vi "RS232c.vi"() -> ()   [LabVIEW 2015]
uses:
  <vilib>/Instr/_visa.llb/VISA Configure Serial Port (Instr).vi
  <instrlib>/Agilent 532XX Series/Public/Data/Low Level/Fetch Measurement (Single).vi
  <instrlib>/Agilent 532XX Series/Agilent 532XX Series.lvlib
panel:
  out "Ph = ADAM-4017, CH3 [ V ]:":string
  out "Ph = ADAM-4017, CH4 [ V ]:":string
  out "Pl = ADAM-4017, CH2 [ V ]:":string
  out "Ph = ADAM-4017, CH1 [ V ]:":string
  out "Read Buffer 1 ADAM-4017: 5":dbl
  out "Read Buffer 1 ADAM-4017: 4":dbl
  out "Write Buffer 1 ADAM-4017: 5":dbl
  out "Write Buffer 1 ADAM-4017: 4":dbl
  out "Read Buffer 1 ADAM-4017: 3":dbl
  out "Write Buffer 1 ADAM-4017: 3":dbl
  out "Read Buffer 1 ADAM-4017: 2":dbl
  out "Write Buffer 1 ADAM-4017: 2":dbl
  out "Tiempo 2":dbl
  in  "stop 2":bool
  in  "Tab Control":enum32{"CONFIGURATION", "ERROR"}(tab)
  out "?":dbl
  out "Humidity[ppm]":dbl
  out "Substance 1[ppm]":dbl
  out "Substance 2[ppm]":dbl
  in  "ENABLE CONFIGURATION":bool
  in  "baud rate (9600)":u32=115200
  in  "data bits (8)":u16=8 min=5 max=8 step=1
  in  "parity (0:none)":u16(ring) items=["None", "Odd", "Even", "Mark", "Space"]
  in  "flow control":u16(ring) items=["None"=0, "XON/XOFF"=1, "RTS/CTS"=2, "DTR/DSR"=4]
  in  "VISA resource name (write)":refnum<visa-resource-name>="COM1"
  in  "stop bits":u16(ring)=10 items=["1.0"=10, "1.5"=15, "2.0"=20]
  in  "Voltios":dbl
  out "output string":string
  out "output string 3":string
  in  "Voltios 2":dbl
  out "output string 4":string
  in  "Voltios 3":dbl
  out "output string 5":string
  in  "Voltios 4":dbl
  in  "VISA resource name":refnum<visa-resource-name>
  in  "Timeout (10000 ms)":u32=10000
  out "Measurement":dbl format="%#_12g"
  out "Canal 4":cluster{dbl[], dbl[]}(graph) caption="Temperatura SAW"
  out "Ph = ADAM-4017, CH1 [ V ]:":string
  out "Ph = ADAM-4017, CH2 [ V ]:":string
  out "Ph = ADAM-4017, CH4 [ V ]:":string
  out "Ph = ADAM-4017, CH5 [ V ]:":string
  out "Write Buffer 1 ADAM-4017:":dbl
  out "Read Buffer 1 ADAM-4017:":dbl
  out "Write Buffer 2 ADAM-4017:":dbl
  out "Read Buffer 2 ADAM-4017:":dbl
  out "Write Buffer 3 ADAM-4017:":dbl
  out "Read Buffer 3 ADAM-4017:":dbl
  out "Read Buffer 4 ADAM-4017:":dbl
  out "Write Buffer 4 ADAM-4017:":dbl
  in  "error in (no error)":errorcluster
  out "error out":errorcluster
  out "VISA resource name out":refnum<visa-resource-name>
  out "Time:":string="00:00:00"
  out "Date:":string="01-01-2010"
  out "bytes written 5":u32=1
  out "bytes written 4":u32=1
  out "bytes written 3":u32=1
  out "bytes written 2":u32=1
  out "output string 2":string
  out "return count":u32
  out "Serial Settings:Number of Bytes at Serial Port":u32
  out "unsigned byte array 2":u8[](array[numeric])
  out "read buffer":string
  out "bytes written":u32=1
  # "WRITE"
  # "Air [ppm]"
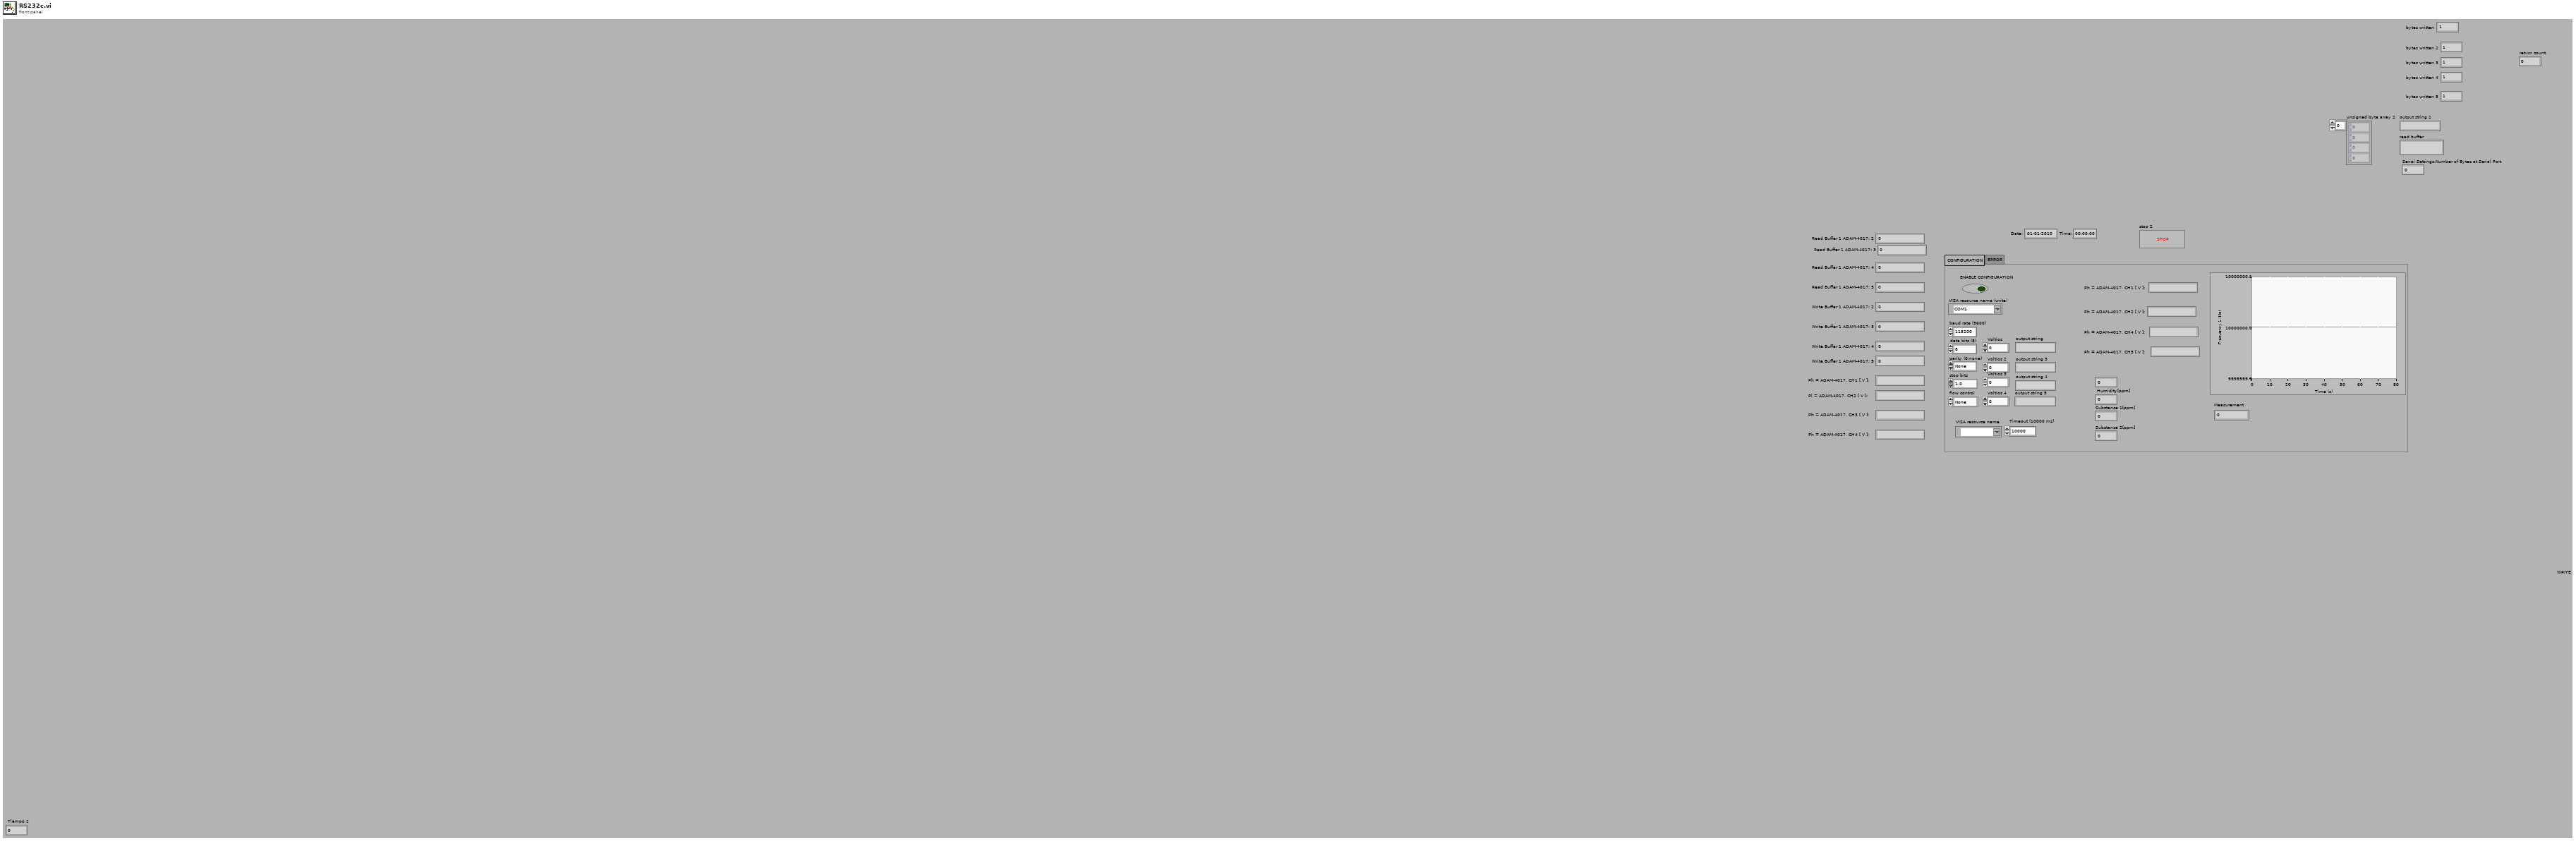
[diagram p1: front panel]
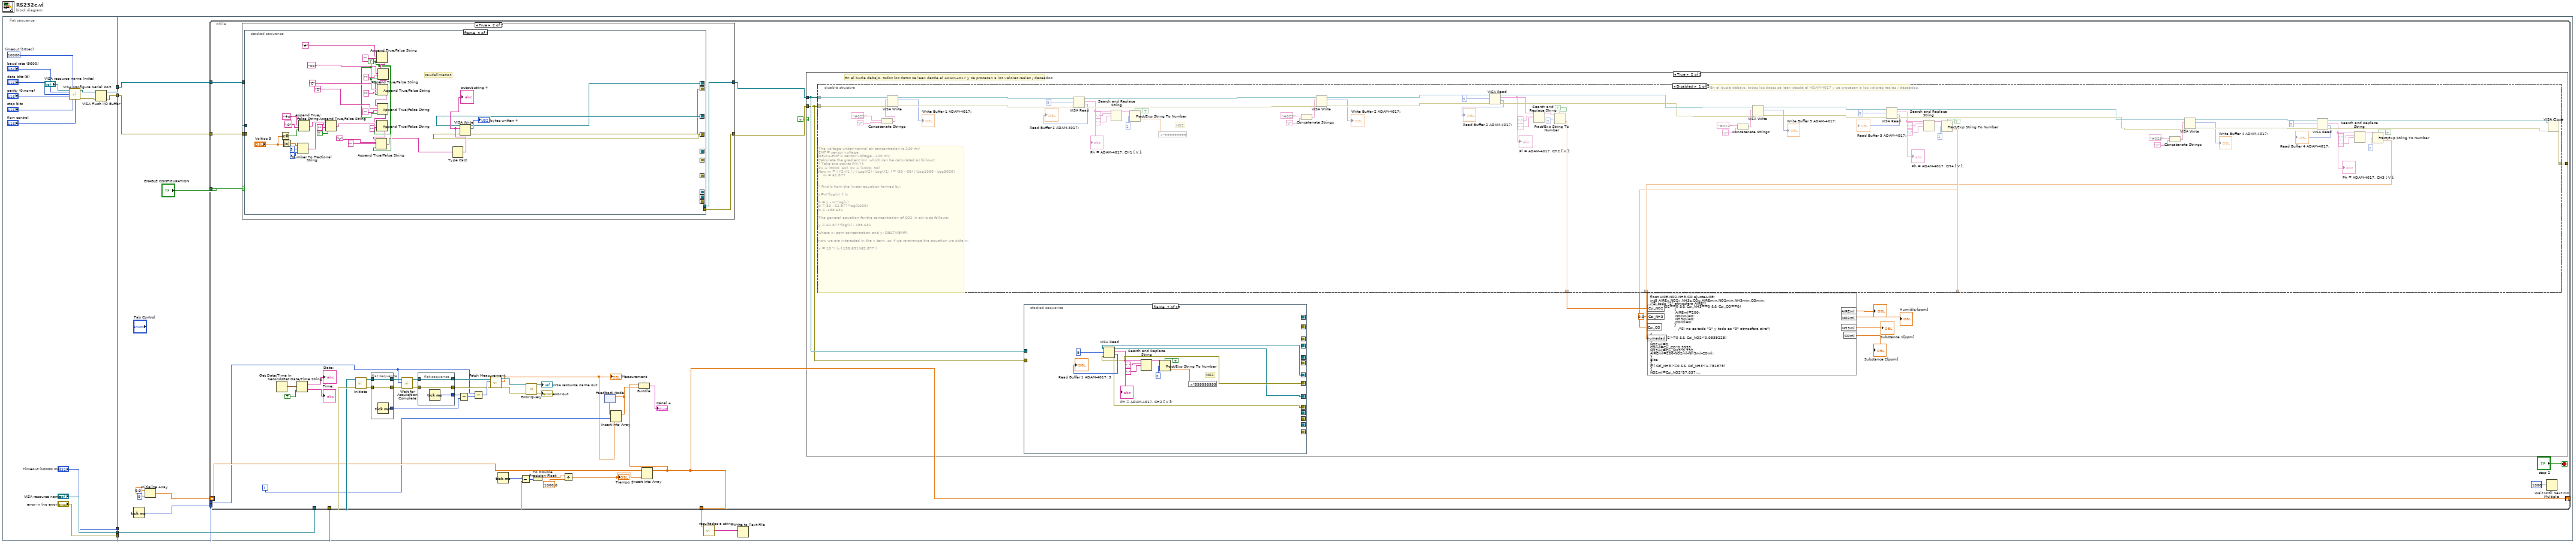
[diagram p0: block diagram]
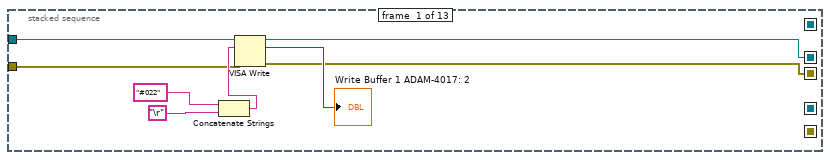
[diagram p4: hidden frame]
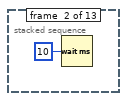
[diagram p5: hidden frame]
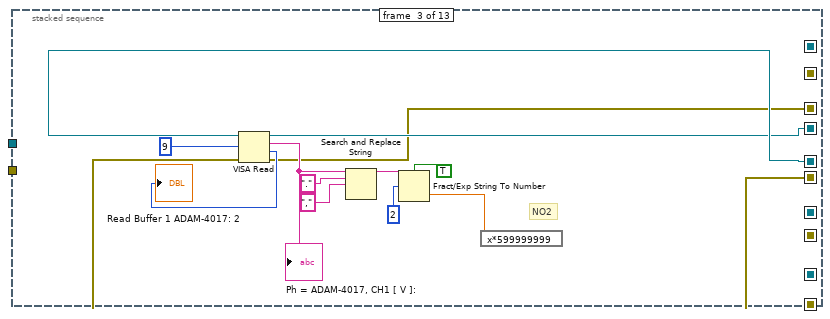
[diagram p6: hidden frame]
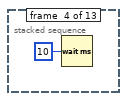
[diagram p7: hidden frame]
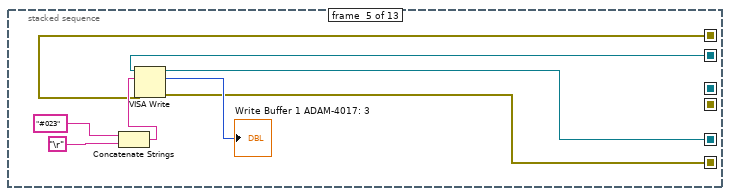
[diagram p8: hidden frame]
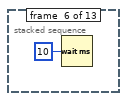
[diagram p9: hidden frame]
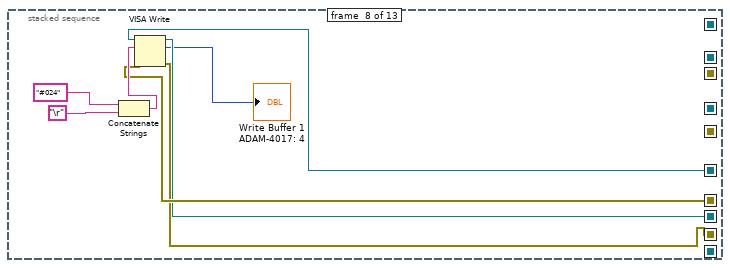
[diagram p10: hidden frame]
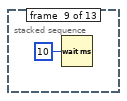
[diagram p11: hidden frame]
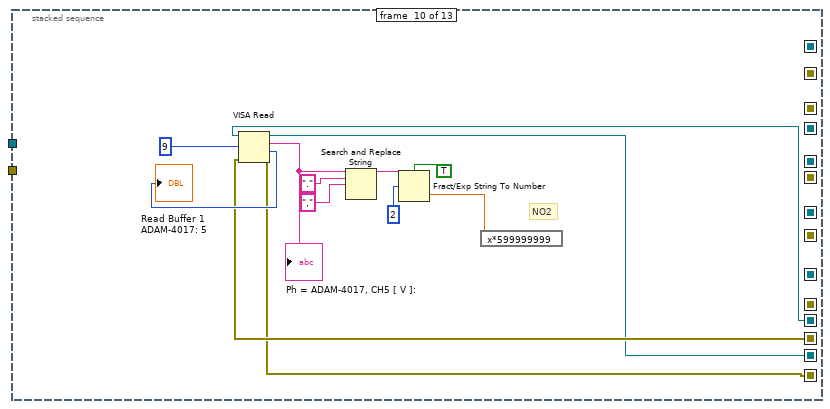
[diagram p12: hidden frame]
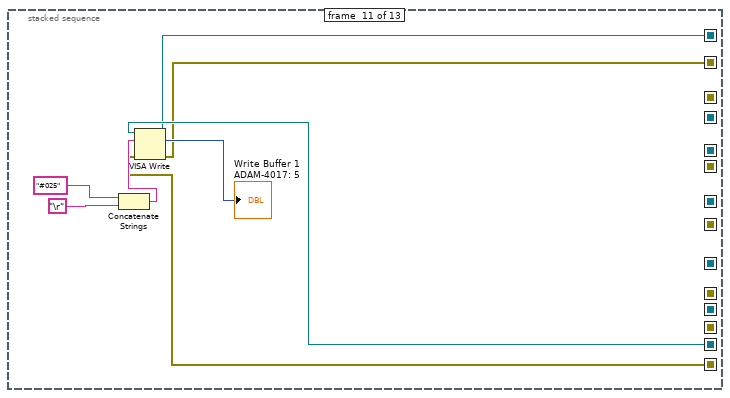
[diagram p13: hidden frame]
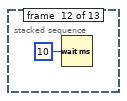
[diagram p14: hidden frame]
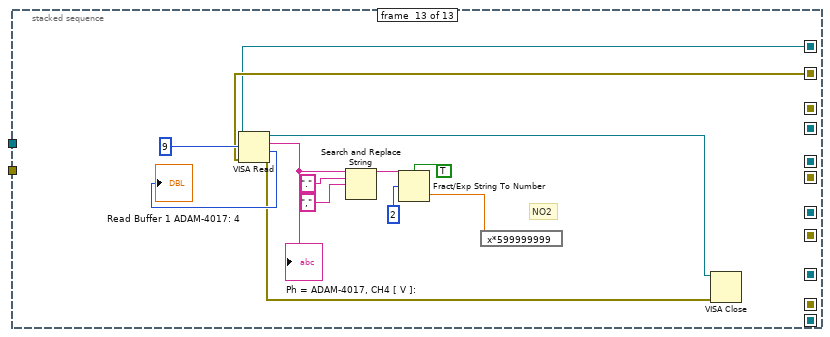
[diagram p15: hidden frame]
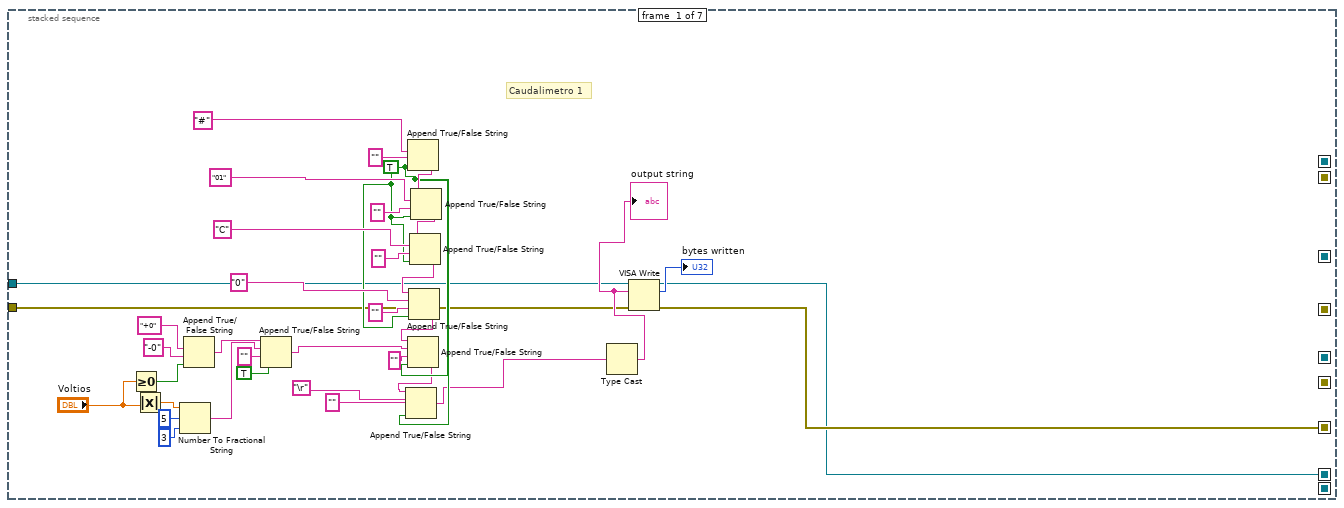
[diagram p17: hidden frame]
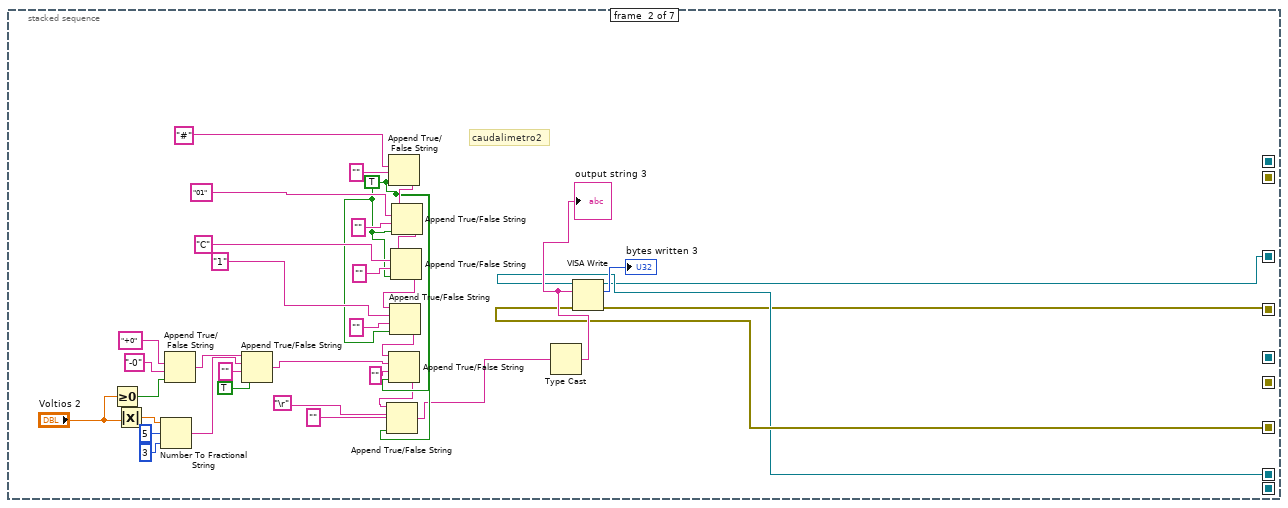
[diagram p18: hidden frame]
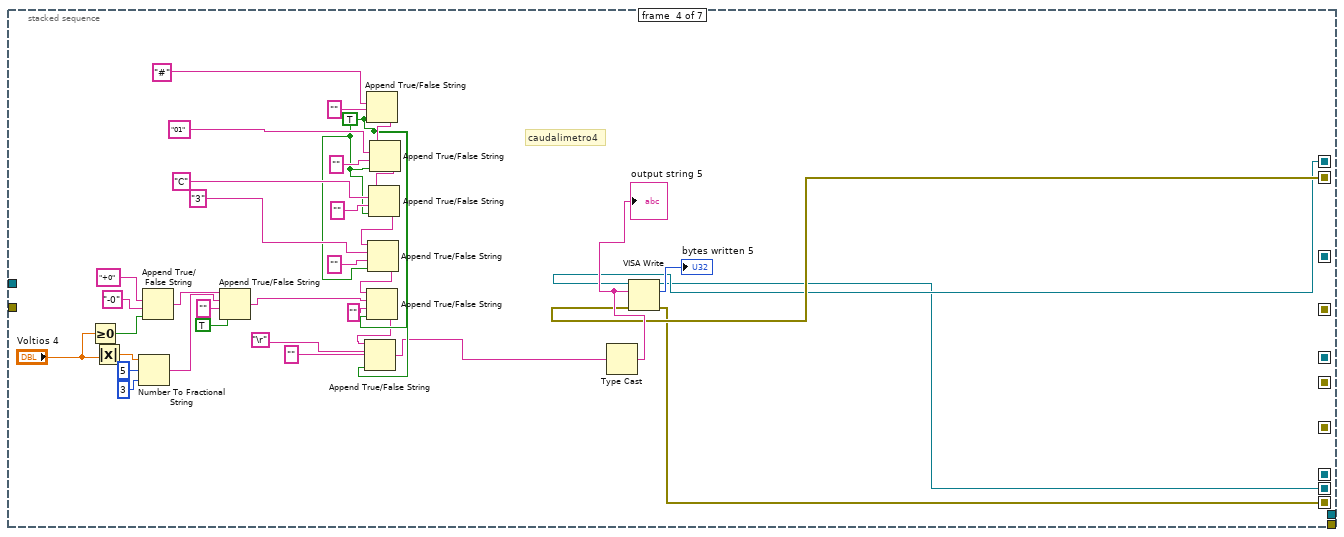
[diagram p19: hidden frame]
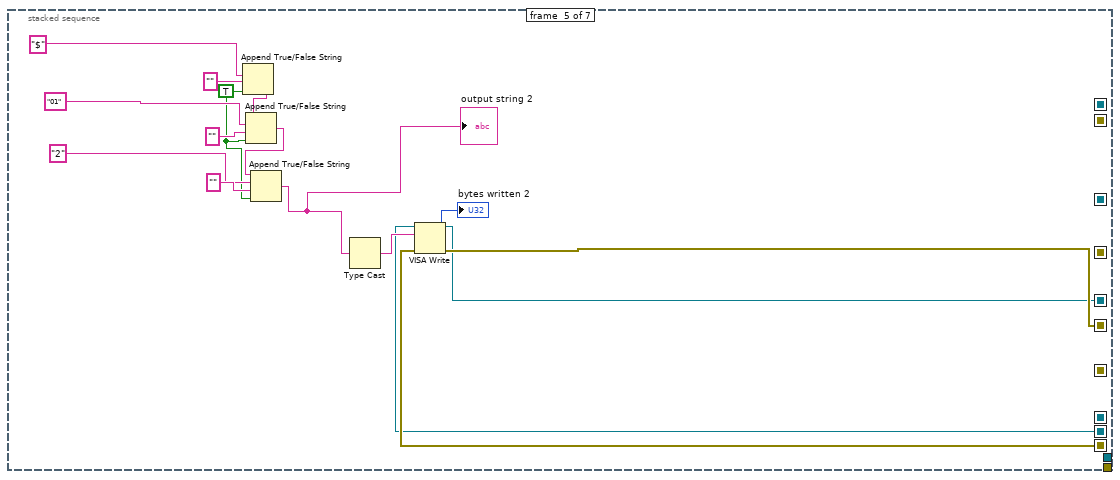
[diagram p20: hidden frame]
diagram:
  n1 = flat-sequence {
    tunnel: [w10] -> w5
    tunnel: [w9] -> w4
    tunnel: ["error in (no error)"] -> w3
    tunnel: ["VISA resource name"] -> w2
    tunnel: ["Timeout (10000 ms)"] -> w1
    tunnel: w5 -> [w31]
    tunnel: w4 -> [w30]
    tunnel: w3 -> [w28]
    tunnel: w2 -> [w27]
    tunnel: w1 -> [w26]
    frame #0 {
      w12 = u32 10000  # timeout (10sec)
      n2 = call-poly "VISA Configure Serial Port"("VISA resource name"="VISA resource name (write)", "timeout (10sec)"=w12, "baud rate (9600)"="baud rate (9600)", "data bits (8)"="data bits (8)", "parity (0:none)"="parity (0:none)", "stop bits (10: 1 bit)"="stop bits", "flow control (0:none)"="flow control") -> ("VISA resource name out"=w18:refnum<visa-resource-name>, "error out"=w19:errorcluster)  [unwired: 7 in]
      n3 = VISA Flush I/O Buffer(VISA resource name=w18, error in (no error)=w19) -> (VISA resource name out=w9:refnum<visa-resource-name>, error out=w10:errorcluster)  [unwired: 1 in]
    }
    frame #1 {
      n4 = Tick Count (ms)() -> (millisecond timer value=w25:u32)
      n5 = Initialize Array(0.0 ("element"), 0 ("dimension size")) -> (w22:dbl[])
      n6 = while {
        tunnel: w31 -> [w75]
        tunnel: w30 -> [w74]
        tunnel: "ENABLE CONFIGURATION" -> [w73]
        tunnel: w28 -> [w47]
        tunnel: w27 -> [w46]
        tunnel: w26 -> [w32]
        shift-right: [w33] -> _
        shift-left: w22 -> [w40]
        tunnel: w25 -> [w39]
        tunnel: [w33] -> w20
        i -> [w37]
        stop <- "stop 2" stop-if-true
        n7 = case shown="True" w73 {
          tunnel: w75 -> [w255 w259]
          tunnel: w74 -> [w254 w258]
          tunnel: [w255 w257] -> w72
          tunnel: [w254 w256] -> w71
          frame False {
          }
          frame True {
            n8 = stacked-sequence {
              seq-local: [w294 _ _ _ _ _ _] -> [_ w299 _ _ _ _ _]
              seq-local: [w293 _ _ _ _ _ _] -> [_ w298 _ _ _ _ _]
              seq-local: [_ _ _ _ w410 _ _] -> [_ _ _ _ _ _ w426]
              seq-local: [_ _ _ _ w409 _ _] -> [_ _ _ _ _ _ w425]
              seq-local: [_ w297 _ _ _ _ _] -> [_ _ w334 _ _ _ _]
              seq-local: [_ w296 _ _ _ _ _] -> [_ _ w335 _ _ _ _]
              seq-local: [_ _ w333 _ _ _ _] -> [_ _ _ w371 _ _ _]
              seq-local: [_ _ w332 _ _ _ _] -> [_ _ _ w370 _ _ _]
              seq-local: [_ _ _ w368 _ _ _] -> [_ _ _ _ w405 _ _]
              seq-local: [_ _ _ w369 _ _ _] -> [_ _ _ _ w406 _ _]
              tunnel: w259 -> [w261 _ _ _ _ _ _]
              tunnel: w258 -> [w260 _ _ _ _ _ _]
              tunnel: [_ _ _ _ _ _ w422] -> w257
              tunnel: [_ _ _ _ _ _ w421] -> w256
              frame #0 {
                w279 = TRUE ("selector")
                # "Caudalimetro 1"
                n9 = Greater Or Equal To 0?(x="Voltios") -> (x >= 0?=w267:bool)
                n10 = Absolute Value(x="Voltios") -> (abs(x)=w265:dbl)
                n11 = Number To Fractional String(number=w265, width (-)=i16 5, precision (6)=i16 3) -> (F-format string=w271:string)  [unwired: 1 in]
                n12 = Append True/False String(1:w267, 2:"-0" ("false string"), 3:"+0") -> (0:w272:string)  [unwired: 1 in]
                n13 = Append True/False String(1:TRUE ("selector"), 2:"" ("false string"), 3:w271, 4:w272) -> (0:w266:string)
                n14 = Append True/False String(1:w279, 2:"" ("false string"), 3:"#") -> (0:w287:string)  [unwired: 1 in]
                n15 = Append True/False String(1:w279, 2:"" ("false string"), 3:"01" ("INI"), 4:w287) -> (0:w286:string)
                n16 = Append True/False String(1:w279, 2:"" ("false string"), 3:"C" ("MASK"), 4:w286) -> (0:w292:string)
                n17 = Append True/False String(1:w279, 2:"" ("false string"), 3:"0" ("Canal"), 4:w292) -> (0:w280:string)
                n18 = Append True/False String(1:w279, 2:"", 3:w266, 4:w280) -> (0:w277:string)
                n19 = Append True/False String(1:w279, 2:"" ("false string"), 3:"\r", 4:w277) -> (0:w263:string)
                n20 = Type Cast(x=w263) -> (*(type *) &x=w262:string)  [unwired: 1 in]
                "output string" <- w262
                n21 = VISA Write(VISA resource name=w260, write buffer=w262, error in (no error)=w261) -> (VISA resource name out=w293:refnum<visa-resource-name>, return count=→"bytes written":u32, error out=w294:errorcluster)
              }
              frame #1 {
                w317 = TRUE ("selector")
                # "caudalimetro2"
                n22 = Greater Or Equal To 0?(x="Voltios 2") -> (x >= 0?=w305:bool)
                n23 = Absolute Value(x="Voltios 2") -> (abs(x)=w303:dbl)
                n24 = Number To Fractional String(number=w303, width (-)=i16 5, precision (6)=i16 3) -> (F-format string=w309:string)  [unwired: 1 in]
                n25 = Append True/False String(1:w305, 2:"-0" ("false string"), 3:"+0") -> (0:w310:string)  [unwired: 1 in]
                n26 = Append True/False String(1:TRUE ("selector"), 2:"" ("false string"), 3:w309, 4:w310) -> (0:w304:string)
                n27 = Append True/False String(1:w317, 2:"" ("false string"), 3:"#") -> (0:w325:string)  [unwired: 1 in]
                n28 = Append True/False String(1:w317, 2:"" ("false string"), 3:"01" ("INI"), 4:w325) -> (0:w324:string)
                n29 = Append True/False String(1:w317, 2:"" ("false string"), 3:"C" ("MASK"), 4:w324) -> (0:w330:string)
                n30 = Append True/False String(1:w317, 2:"" ("false string"), 3:"1" ("Canal 2"), 4:w330) -> (0:w318:string)
                n31 = Append True/False String(1:w317, 2:"", 3:w304, 4:w318) -> (0:w315:string)
                n32 = Append True/False String(1:w317, 2:"" ("false string"), 3:"\r", 4:w315) -> (0:w301:string)
                n33 = Type Cast(x=w301) -> (*(type *) &x=w300:string)  [unwired: 1 in]
                "output string 3" <- w300
                n34 = VISA Write(VISA resource name=w298, write buffer=w300, error in (no error)=w299) -> (VISA resource name out=w296:refnum<visa-resource-name>, return count=→"bytes written 3":u32, error out=w297:errorcluster)
              }
              frame #2 {
                w353 = TRUE ("selector")
                # "caudalimetro3"
                n35 = Greater Or Equal To 0?(x="Voltios 3") -> (x >= 0?=w341:bool)
                n36 = Absolute Value(x="Voltios 3") -> (abs(x)=w339:dbl)
                n37 = Number To Fractional String(number=w339, width (-)=i16 5, precision (6)=i16 3) -> (F-format string=w345:string)  [unwired: 1 in]
                n38 = Append True/False String(1:w341, 2:"-0" ("false string"), 3:"+0") -> (0:w346:string)  [unwired: 1 in]
                n39 = Append True/False String(1:TRUE ("selector"), 2:"" ("false string"), 3:w345, 4:w346) -> (0:w340:string)
                n40 = Append True/False String(1:w353, 2:"" ("false string"), 3:"#") -> (0:w361:string)  [unwired: 1 in]
                n41 = Append True/False String(1:w353, 2:"" ("false string"), 3:"01" ("INI"), 4:w361) -> (0:w360:string)
                n42 = Append True/False String(1:w353, 2:"" ("false string"), 3:"C" ("MASK"), 4:w360) -> (0:w366:string)
                n43 = Append True/False String(1:w353, 2:"" ("false string"), 3:"2" ("Canal 3"), 4:w366) -> (0:w354:string)
                n44 = Append True/False String(1:w353, 2:"", 3:w340, 4:w354) -> (0:w351:string)
                n45 = Append True/False String(1:w353, 2:"" ("false string"), 3:"\r", 4:w351) -> (0:w337:string)
                n46 = Type Cast(x=w337) -> (*(type *) &x=w336:string)  [unwired: 1 in]
                "output string 4" <- w336
                n47 = VISA Write(VISA resource name=w335, write buffer=w336, error in (no error)=w334) -> (VISA resource name out=w332:refnum<visa-resource-name>, return count=→"bytes written 4":u32, error out=w333:errorcluster)
              }
              frame #3 {
                w389 = TRUE ("selector")
                # "caudalimetro4"
                n48 = Greater Or Equal To 0?(x="Voltios 4") -> (x >= 0?=w377:bool)
                n49 = Absolute Value(x="Voltios 4") -> (abs(x)=w375:dbl)
                n50 = Number To Fractional String(number=w375, width (-)=i16 5, precision (6)=i16 3) -> (F-format string=w381:string)  [unwired: 1 in]
                n51 = Append True/False String(1:w377, 2:"-0" ("false string"), 3:"+0") -> (0:w382:string)  [unwired: 1 in]
                n52 = Append True/False String(1:TRUE ("selector"), 2:"" ("false string"), 3:w381, 4:w382) -> (0:w376:string)
                n53 = Append True/False String(1:w389, 2:"" ("false string"), 3:"#") -> (0:w397:string)  [unwired: 1 in]
                n54 = Append True/False String(1:w389, 2:"" ("false string"), 3:"01" ("INI"), 4:w397) -> (0:w396:string)
                n55 = Append True/False String(1:w389, 2:"" ("false string"), 3:"C" ("MASK"), 4:w396) -> (0:w402:string)
                n56 = Append True/False String(1:w389, 2:"" ("false string"), 3:"3" ("Canal 4"), 4:w402) -> (0:w390:string)
                n57 = Append True/False String(1:w389, 2:"", 3:w376, 4:w390) -> (0:w387:string)
                n58 = Append True/False String(1:w389, 2:"" ("false string"), 3:"\r", 4:w387) -> (0:w373:string)
                n59 = Type Cast(x=w373) -> (*(type *) &x=w372:string)  [unwired: 1 in]
                "output string 5" <- w372
                n60 = VISA Write(VISA resource name=w370, write buffer=w372, error in (no error)=w371) -> (VISA resource name out=w368:refnum<visa-resource-name>, return count=→"bytes written 5":u32, error out=w369:errorcluster)
              }
              frame #4 {
                w408 = TRUE ("selector")
                n61 = Append True/False String(1:w408, 2:"" ("false string"), 3:"$") -> (0:w415:string)  [unwired: 1 in]
                n62 = Append True/False String(1:w408, 2:"" ("false string"), 3:"01" ("INI"), 4:w415) -> (0:w414:string)
                n63 = Append True/False String(1:w408, 2:"" ("false string"), 3:"2" ("MASK"), 4:w414) -> (0:w404:string)
                "output string 2" <- w404
                n64 = Type Cast(x=w404) -> (*(type *) &x=w407:string)  [unwired: 1 in]
                n65 = VISA Write(VISA resource name=w405, write buffer=w407, error in (no error)=w406) -> (VISA resource name out=w409:refnum<visa-resource-name>, return count=→"bytes written 2":u32, error out=w410:errorcluster)
              }
              frame #5 {
                n66 = Wait (ms)(milliseconds to wait=u32 1000) -> ()  [unwired: 1 out]
              }
              frame #6 {
                n67 = property class="Instr"(reference=w425, error in=w426) -> (reference out=w431:refnum<visa-resource-name>, error out=w430:errorcluster, "Bytes at Port"=w429:u32)
                "Serial Settings:Number of Bytes at Serial Port" <- w429
                n68 = VISA Read(VISA resource name=w431, byte count=w429, error in (no error)=w430) -> (VISA resource name out=w421:refnum<visa-resource-name>, read buffer=w424:string, return count=→"return count":u32, error out=w422:errorcluster)
                n69 = String To Byte Array(string=w424) -> (unsigned byte array=→"unsigned byte array 2":u8[])
                n70 = Type Cast(x=w424) -> (*(type *) &x=→"read buffer":string)  [unwired: 1 in]
              }
            }
          }
        }
        n71 = Get Date/Time In Seconds() -> (seconds since 1Jan1904=w67:timestamp)
        n72 = Get Date/Time String(seconds (now)=w67, want seconds? (F)=TRUE) -> (date string=→"Date:":string, time string=→"Time:":string)  [unwired: 1 in]
        n73 = call <instrlib>:"Initiate.vi"("error in (no error)"=w47, "VISA resource name"=w46) -> ("error out"=w59:errorcluster, "VISA resource name out"=w60:refnum<visa-resource-name>)  [unwired: 8 out]
        n74 = flat-sequence {
          tunnel: [w81] -> w56
          tunnel: w60 -> [w81]
          tunnel: [w80] -> w57
          tunnel: w59 -> [w80]
          tunnel: [w79] -> w58
          frame #0 {
            n75 = Tick Count (ms)() -> (millisecond timer value=w79:u32)
          }
        }
        n76 = call <instrlib>:"Wait for Acquisition Complete.vi"("error in (no error)"=w57, "Maximum Time (10000 ms)"=w32, "VISA resource name"=w56) -> ("error out"=w54:errorcluster, "VISA resource name out"=w55:refnum<visa-resource-name>)  [unwired: 1 in, 6 out]
        n77 = flat-sequence {
          tunnel: [w78] -> w50
          tunnel: w55 -> [w78]
          tunnel: [w77] -> w51
          tunnel: w54 -> [w77]
          tunnel: [w76] -> w53
          frame #0 {
            n78 = Tick Count (ms)() -> (millisecond timer value=w76:u32)
          }
        }
        n79 = Subtract(x=w53, y=w58) -> (x-y=w61:u32)
        n80 = Subtract(x=w32, y=w61) -> (x-y=w52:u32)
        n81 = call-poly <instrlib>:"Fetch Measurement.vi"("error in (no error)"=w51, "Timeout (10000 ms)"=w52, "VISA resource name"=w50) -> ("error out"=w48:errorcluster, "Measurement"=w35:dbl, "VISA resource name out"=w49:refnum<visa-resource-name>)  [unwired: 6 out]
        "Measurement" <- w35
        n82 = Tick Count (ms)() -> (millisecond timer value=w45:u32)
        n83 = Subtract(x=w45, y=w39) -> (x-y=w43:u32)
        n84 = call <instrlib>:"Error Query.vi"("error in (no error)"=w48, "VISA resource name"=w49) -> ("error out"=→"error out":errorcluster, "VISA resource name out"=→"VISA resource name out":refnum<visa-resource-name>)  [unwired: 8 out]
        n85 = To Double Precision Float(number=w43) -> (double precision float=w42:dbl)
        n86 = Divide(x=w42, y=1000.0 ("x/y")) -> (x/y=w41:dbl)
        "Tiempo 2" <- w41
        n87 = feedback #1() -> (w38:dbl[])  [unwired: 1 in]
        n88 = Insert Into Array(array=w38, index=w37, new element=w35) -> (w36:dbl[])
        n89 = feedback-in #1(w36) -> ()
        n90 = Insert Into Array(array=w40, new element=w41) -> (w33:dbl[])  [unwired: 1 in]
        n91 = Bundle(w33, w36) -> (→"Canal 4":cluster{dbl[], dbl[]})  [unwired: 1 in]
        n92 = case shown="True" TRUE {
          tunnel: w72 -> [w82 w83]
          tunnel: w71 -> [_ w84]
          tunnel: [w82 w93] -> _
          frame False {
          }
          frame True {
            # "En el bucle debajo, todos los datos se leen desde el ADAM-4017 y se procesan a los valores reales / deseados."
            n93 = disable-structure shown="Disabled" {
              disable-tunnel: [w164 _] -> w93
              disable-tunnel: [w147 _] -> w92
              disable-tunnel: [w146 _] -> w91
              disable-tunnel: [w145 _] -> w90
              disable-tunnel: w83 -> [w95 _]
              disable-tunnel: w84 -> [w94 _]
              frame Disabled {
                # "NO2"
                # "The voltage under normal air concentration is 220 mV\nEMF = sensor voltage\nDELTA-EMF = sensor voltage - 220 mV\nCalculate the gradient (m), which can be calculated as follows:\n* Take two points P(X,Y):\nP1 = (3000, 60), P2 = (1000, 30)\nNow m = ( Y2-Y1 ) / ( Log(X2) - Log(X1) ) = (30 - 60) / (Log1000 - Log3000)\n: . m = 62.877\n\n\n* Find b from the linear equation formed by:\n\ny=m*log(x) + b\n\nb = y - m*log(x)\nb = 30 - 62.877*log(1000)\nb = -158.631\n\nThe general equation for the concentration of CO2 in air is as follows:\n\ny = 62.877*log(x) - 158.631\n\nwhere x: ppm concentration and y: DELTA(EMF).\n\nnow we are interested in the x term, so if we re-arrange the equation we obtain:\n\nx = 10^( (y+158.631)/62.877 )"
                # "En el bucle debajo, todos los datos se leen desde el ADAM-4017 y se procesan a los valores reales / deseados."
                n94 = Concatenate Strings("#022" ("String"), "\r") -> (w142:string)
                n95 = VISA Write(VISA resource name=w94, write buffer=w142, error in (no error)=w95) -> (VISA resource name out=w163:refnum<visa-resource-name>, return count=→"Write Buffer 1 ADAM-4017:":u32, error out=w162:errorcluster)
                n96 = VISA Read(VISA resource name=w163, byte count=9, error in (no error)=w162) -> (VISA resource name out=w158:refnum<visa-resource-name>, read buffer=w133:string, return count=→"Read Buffer 1 ADAM-4017:":u32, error out=w159:errorcluster)
                "Ph = ADAM-4017, CH1 [ V ]:" <- w133
                n97 = Search and Replace String(input string=w133, search string=".", replace string="," ("replace string (\"\")")) -> (result string=w134:string)  [unwired: 5 in, 3 out]
                n98 = Fract/Exp String To Number(use system decimal point (T)=TRUE, string=w134, offset=2) -> (number=w132:dbl)  [unwired: 1 in, 1 out]
                n99 = expression code="x*599999999"(w132) -> ()  [unwired: 1 out]
                n100 = Concatenate Strings("#023" ("String"), "\r") -> (w129:string)
                n101 = VISA Write(VISA resource name=w158, write buffer=w129, error in (no error)=w159) -> (VISA resource name out=w161:refnum<visa-resource-name>, return count=→"Write Buffer 2 ADAM-4017:":u32, error out=w160:errorcluster)
                n102 = VISA Read(VISA resource name=w161, byte count=9, error in (no error)=w160) -> (VISA resource name out=w155:refnum<visa-resource-name>, read buffer=w120:string, return count=→"Read Buffer 2 ADAM-4017:":u32, error out=w154:errorcluster)
                "Pl = ADAM-4017, CH2 [ V ]:" <- w120
                n103 = Search and Replace String(input string=w120, search string=".", replace string="," ("replace string (\"\")")) -> (result string=w124:string)  [unwired: 5 in, 3 out]
                n104 = Fract/Exp String To Number(use system decimal point (T)=TRUE, string=w124, offset=2) -> (number=w147:dbl)  [unwired: 1 in, 1 out]
                n105 = Concatenate Strings("#024" ("String"), "\r") -> (w117:string)
                n106 = VISA Write(VISA resource name=w155, write buffer=w117, error in (no error)=w154) -> (VISA resource name out=w157:refnum<visa-resource-name>, return count=→"Write Buffer 3 ADAM-4017:":u32, error out=w156:errorcluster)
                n107 = VISA Read(VISA resource name=w157, byte count=9, error in (no error)=w156) -> (VISA resource name out=w151:refnum<visa-resource-name>, read buffer=w108:string, return count=→"Read Buffer 3 ADAM-4017:":u32, error out=w150:errorcluster)
                "Ph = ADAM-4017, CH4 [ V ]:" <- w108
                n108 = Search and Replace String(input string=w108, search string=".", replace string="," ("replace string (\"\")")) -> (result string=w109:string)  [unwired: 5 in, 3 out]
                n109 = Fract/Exp String To Number(use system decimal point (T)=TRUE, string=w109, offset=2) -> (number=w146:dbl)  [unwired: 1 in, 1 out]
                n110 = Concatenate Strings("#025" ("String"), "\r") -> (w105:string)
                n111 = VISA Write(VISA resource name=w151, write buffer=w105, error in (no error)=w150) -> (VISA resource name out=w148:refnum<visa-resource-name>, return count=→"Write Buffer 4 ADAM-4017:":u32, error out=w149:errorcluster)
                n112 = VISA Read(VISA resource name=w148, byte count=9, error in (no error)=w149) -> (VISA resource name out=w152:refnum<visa-resource-name>, read buffer=w96:string, return count=→"Read Buffer 4 ADAM-4017:":u32, error out=w153:errorcluster)
                "Ph = ADAM-4017, CH3 [ V ]:" <- w96
                n113 = Search and Replace String(input string=w96, search string=".", replace string="," ("replace string (\"\")")) -> (result string=w97:string)  [unwired: 5 in, 3 out]
                n114 = Fract/Exp String To Number(use system decimal point (T)=TRUE, string=w97, offset=2) -> (number=w145:dbl)  [unwired: 1 in, 1 out]
                n115 = VISA Close(VISA resource name=w152, error in (no error)=w153) -> (error out=w164:errorcluster)
              }
              frame Enabled {
              }
            }
            n116 = stacked-sequence {
              seq-local: [w165 _ _ _ _ _ _ _ _ _ _ _ _] -> [_ _ w176 _ _ _ _ _ _ _ _ _ _]
              seq-local: [w166 _ _ _ _ _ _ _ _ _ _ _ _] -> [_ _ w177 _ _ _ _ _ _ _ _ _ _]
              seq-local: [_ _ w175 _ _ _ _ _ _ _ _ _ _] -> [_ _ _ _ w190 _ _ _ _ _ _ _ _]
              seq-local: [_ _ w174 _ _ _ _ _ _ _ _ _ _] -> [_ _ _ _ w191 _ _ _ _ _ _ _ _]
              seq-local: [_ _ _ _ w189 _ _ _ _ _ _ _ _] -> [_ _ _ _ _ _ w200 _ _ _ _ _ _]
              seq-local: [_ _ _ _ w188 _ _ _ _ _ _ _ _] -> [_ _ _ _ _ _ w199 _ _ _ _ _ _]
              seq-local: [_ _ _ _ _ _ w198 _ _ _ _ _ _] -> [_ _ _ _ _ _ _ w214 _ _ _ _ _]
              seq-local: [_ _ _ _ _ _ w197 _ _ _ _ _ _] -> [_ _ _ _ _ _ _ w213 _ _ _ _ _]
              seq-local: [_ _ _ _ _ _ _ w212 _ _ _ _ _] -> [_ _ _ _ _ _ _ _ _ w222 _ _ _]
              seq-local: [_ _ _ _ _ _ _ w211 _ _ _ _ _] -> [_ _ _ _ _ _ _ _ _ w221 _ _ _]
              seq-local: [_ _ _ _ _ _ _ _ _ w219 _ _ _] -> [_ _ _ _ _ _ _ _ _ _ w234 _ _]
              seq-local: [_ _ _ _ _ _ _ _ _ w220 _ _ _] -> [_ _ _ _ _ _ _ _ _ _ w235 _ _]
              seq-local: [_ _ _ _ _ _ _ _ _ _ w232 _ _] -> [_ _ _ _ _ _ _ _ _ _ _ _ w241]
              seq-local: [_ _ _ _ _ _ _ _ _ _ w233 _ _] -> [_ _ _ _ _ _ _ _ _ _ _ _ w242]
              tunnel: w84 -> [w168 _ _ _ _ _ _ _ _ _ _ _ _]
              tunnel: w83 -> [w167 _ _ _ _ _ _ _ _ _ _ _ _]
              frame #0 {
                n117 = Concatenate Strings("#022" ("String"), "\r") -> (w170:string)
                n118 = VISA Write(VISA resource name=w168, write buffer=w170, error in (no error)=w167) -> (VISA resource name out=w166:refnum<visa-resource-name>, return count=→"Write Buffer 1 ADAM-4017: 2":u32, error out=w165:errorcluster)
              }
              frame #1 {
                n119 = Wait (ms)(milliseconds to wait=u32 10) -> ()  [unwired: 1 out]
              }
              frame #2 {
                # "NO2"
                n120 = VISA Read(VISA resource name=w177, byte count=9, error in (no error)=w176) -> (VISA resource name out=w175:refnum<visa-resource-name>, read buffer=w179:string, return count=→"Read Buffer 1 ADAM-4017: 2":u32, error out=w174:errorcluster)
                "Ph = ADAM-4017, CH1 [ V ]:" <- w179
                n121 = Search and Replace String(input string=w179, search string=".", replace string="," ("replace string (\"\")")) -> (result string=w180:string)  [unwired: 5 in, 3 out]
                n122 = Fract/Exp String To Number(use system decimal point (T)=TRUE, string=w180, offset=2) -> (number=w178:dbl)  [unwired: 1 in, 1 out]
                n123 = expression code="x*599999999"(w178) -> ()  [unwired: 1 out]
              }
              frame #3 {
                n124 = Wait (ms)(milliseconds to wait=u32 10) -> ()  [unwired: 1 out]
              }
              frame #4 {
                n125 = Concatenate Strings("#023" ("String"), "\r") -> (w193:string)
                n126 = VISA Write(VISA resource name=w190, write buffer=w193, error in (no error)=w191) -> (VISA resource name out=w189:refnum<visa-resource-name>, return count=→"Write Buffer 1 ADAM-4017: 3":u32, error out=w188:errorcluster)
              }
              frame #5 {
                n127 = Wait (ms)(milliseconds to wait=u32 10) -> ()  [unwired: 1 out]
              }
              frame #6 {
                # "NO2"
                n128 = VISA Read(VISA resource name=w200, byte count=9, error in (no error)=w199) -> (VISA resource name out=w198:refnum<visa-resource-name>, read buffer=w202:string, return count=→"Read Buffer 1 ADAM-4017: 3":u32, error out=w197:errorcluster)
                "Ph = ADAM-4017, CH2 [ V ]:" <- w202
                n129 = Search and Replace String(input string=w202, search string=".", replace string="," ("replace string (\"\")")) -> (result string=w203:string)  [unwired: 5 in, 3 out]
                n130 = Fract/Exp String To Number(use system decimal point (T)=TRUE, string=w203, offset=2) -> (number=w201:dbl)  [unwired: 1 in, 1 out]
                n131 = expression code="x*599999999"(w201) -> ()  [unwired: 1 out]
              }
              frame #7 {
                n132 = Concatenate Strings("#024" ("String"), "\r") -> (w215:string)
                n133 = VISA Write(VISA resource name=w214, write buffer=w215, error in (no error)=w213) -> (VISA resource name out=w212:refnum<visa-resource-name>, return count=→"Write Buffer 1 ADAM-4017: 4":u32, error out=w211:errorcluster)
              }
              frame #8 {
                n134 = Wait (ms)(milliseconds to wait=u32 10) -> ()  [unwired: 1 out]
              }
              frame #9 {
                # "NO2"
                n135 = VISA Read(VISA resource name=w222, byte count=9, error in (no error)=w221) -> (VISA resource name out=w219:refnum<visa-resource-name>, read buffer=w224:string, return count=→"Read Buffer 1 ADAM-4017: 5":u32, error out=w220:errorcluster)
                "Ph = ADAM-4017, CH5 [ V ]:" <- w224
                n136 = Search and Replace String(input string=w224, search string=".", replace string="," ("replace string (\"\")")) -> (result string=w225:string)  [unwired: 5 in, 3 out]
                n137 = Fract/Exp String To Number(use system decimal point (T)=TRUE, string=w225, offset=2) -> (number=w223:dbl)  [unwired: 1 in, 1 out]
                n138 = expression code="x*599999999"(w223) -> ()  [unwired: 1 out]
              }
              frame #10 {
                n139 = Concatenate Strings("#025" ("String"), "\r") -> (w237:string)
                n140 = VISA Write(VISA resource name=w234, write buffer=w237, error in (no error)=w235) -> (VISA resource name out=w232:refnum<visa-resource-name>, return count=→"Write Buffer 1 ADAM-4017: 5":u32, error out=w233:errorcluster)
              }
              frame #11 {
                n141 = Wait (ms)(milliseconds to wait=u32 10) -> ()  [unwired: 1 out]
              }
              frame #12 {
                # "NO2"
                n142 = VISA Read(VISA resource name=w241, byte count=9, error in (no error)=w242) -> (VISA resource name out=w243:refnum<visa-resource-name>, read buffer=w246:string, return count=→"Read Buffer 1 ADAM-4017: 4":u32, error out=w244:errorcluster)
                "Ph = ADAM-4017, CH4 [ V ]:" <- w246
                n143 = Search and Replace String(input string=w246, search string=".", replace string="," ("replace string (\"\")")) -> (result string=w247:string)  [unwired: 5 in, 3 out]
                n144 = Fract/Exp String To Number(use system decimal point (T)=TRUE, string=w247, offset=2) -> (number=w245:dbl)  [unwired: 1 in, 1 out]
                n145 = expression code="x*599999999"(w245) -> ()  [unwired: 1 out]
                n146 = VISA Close(VISA resource name=w243, error in (no error)=w244) -> ()  [unwired: 1 out]
              }
            }
            n147 = formula code="float AIRE,NO2,NH3,CO,ajusteAIRE;\nint8 AIREx,NO2y,NH3z,COu,AIREmin,NO2min,NH3min,COmin;\n/*Si todo \"1\" atmosfera AIRE*/\nif (Csi_NO2==0 && Csi_NH3==0 && Csi_CO==0)\n                    {\n                     AIREml=200;                 \n                     NO2ml=0;\n                     NH3ml=0;\n                     COml=0;\n                    }\n else                /*Si no es todo \"1\" y todo es \"0\" atmosfera aire*/\n                   \n{\nif( Csi_NO2>=0 && Csi_NO2<0.0339225)\n{\nNO2ml=0;\nCOml=Csi_CO*0.3955;\nNH3ml=Csi_NH3*0.752;\nAIREml=200-NO2ml-NH3ml-COml;\n}\nelse\n{\nif ( Csi_NH3>=0 && Csi_NH3<1.781875)\n{\nNO2ml=Csi_NO2*37.037;\nCOml=Csi_CO*0.3955;\nNH3ml=0;\nAIREml=200-NO2ml-NH3ml-COml;\n}\nelse\n{\nif ( Csi_CO>=0 && Csi_CO<1.40375)\n{\nNO2ml=Csi_NO2*37.037;\nCOml=0;\nNH3ml=Csi_NH3*0.752;\nAIREml=200-NO2ml-NH3ml-COml;\n}\nelse\n{\n/*Asignacion de flujos*/\nNO2ml=Csi_NO2*37.037;\nCOml=Csi_CO*0.3955;\nNH3ml=Csi_NH3*0.752;\nAIREml=200-NO2ml-NH3ml-COml;                \n}\n}\n}\n}"("Csi_NH3"=0.0 ("input variable"), "Csi_NO2"=w92, "Csi_CO"=w91, "humedad"=w90) -> ("COml"=→"Substance 2[ppm]":dbl, "NH3ml"=→"Substance 1[ppm]":dbl, "NO2ml"=→"Humidity[ppm]":dbl, "AIREml"=→"?":dbl)
          }
        }
        n148 = Wait Until Next ms Multiple(millisecond multiple=1000) -> ()  [unwired: 1 out]
      }
      n149 = call "resultados a string.vi"("Array"=w20) -> ("concatenated string"=w21:string)  [unwired: 10 in]
      n150 = Write to Text File(text=w21) -> ()  [unwired: 3 in, 3 out]
    }
  }
